vi "file list - sort.vi"(10 "temperature array IN":dbl[](array[numeric]), 11 "path array IN":T1[](array[typedef])) -> (0 "timestamp OUT":dbl[](array[numeric]), 2 "temperatures OUT":dbl[](array[numeric]), 3 "sweep file name array OUT":T1[](array[typedef]))   [LabVIEW 2010]
uses:
  sweep file name.ctl
panel:
  in  "dummy 2":T1={"temperature"=0.0, "temperature str"="", "file path"=path "/snowfall/Users/arcadi/Desktop/Ultrasound/Experiment/YBCO_4/Round1/Sweep12/June_2011/062511/221.16400K_300_3100_001_062511.dat", "last mod"=timestamp(0 s since 1904-01-01), "file name str"="", "mod time(min)"=0.0}
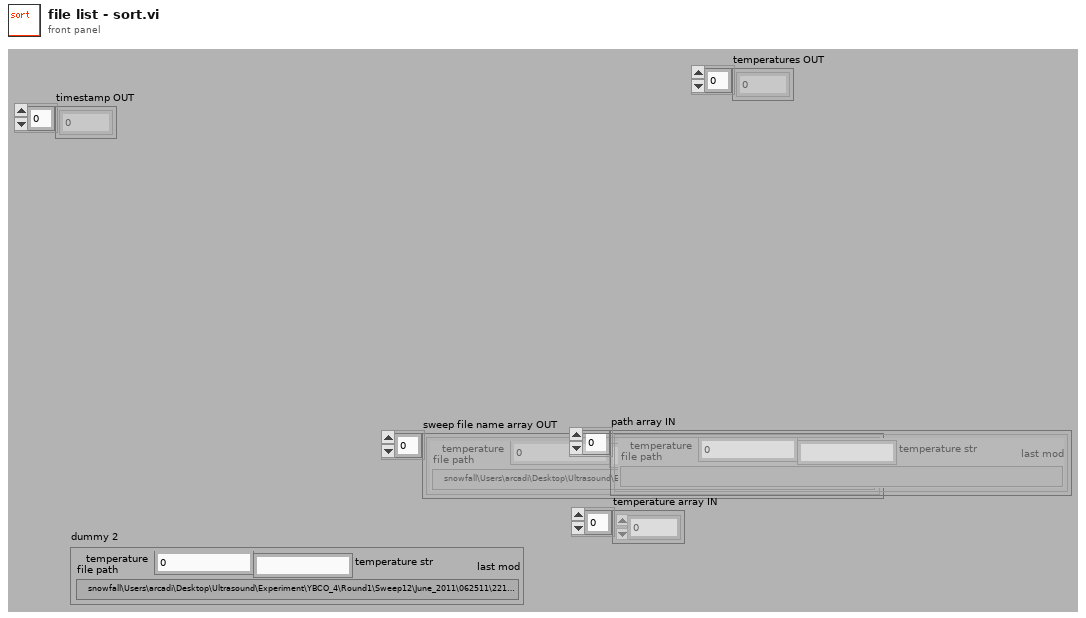
[diagram p1: front panel]
types:
  T1 = typedef "sweep file name.ctl" = cluster{"temperature":dbl, "temperature str":string, "file path":path, "last mod":timestamp, "file name str":string, "mod time(min)":dbl}
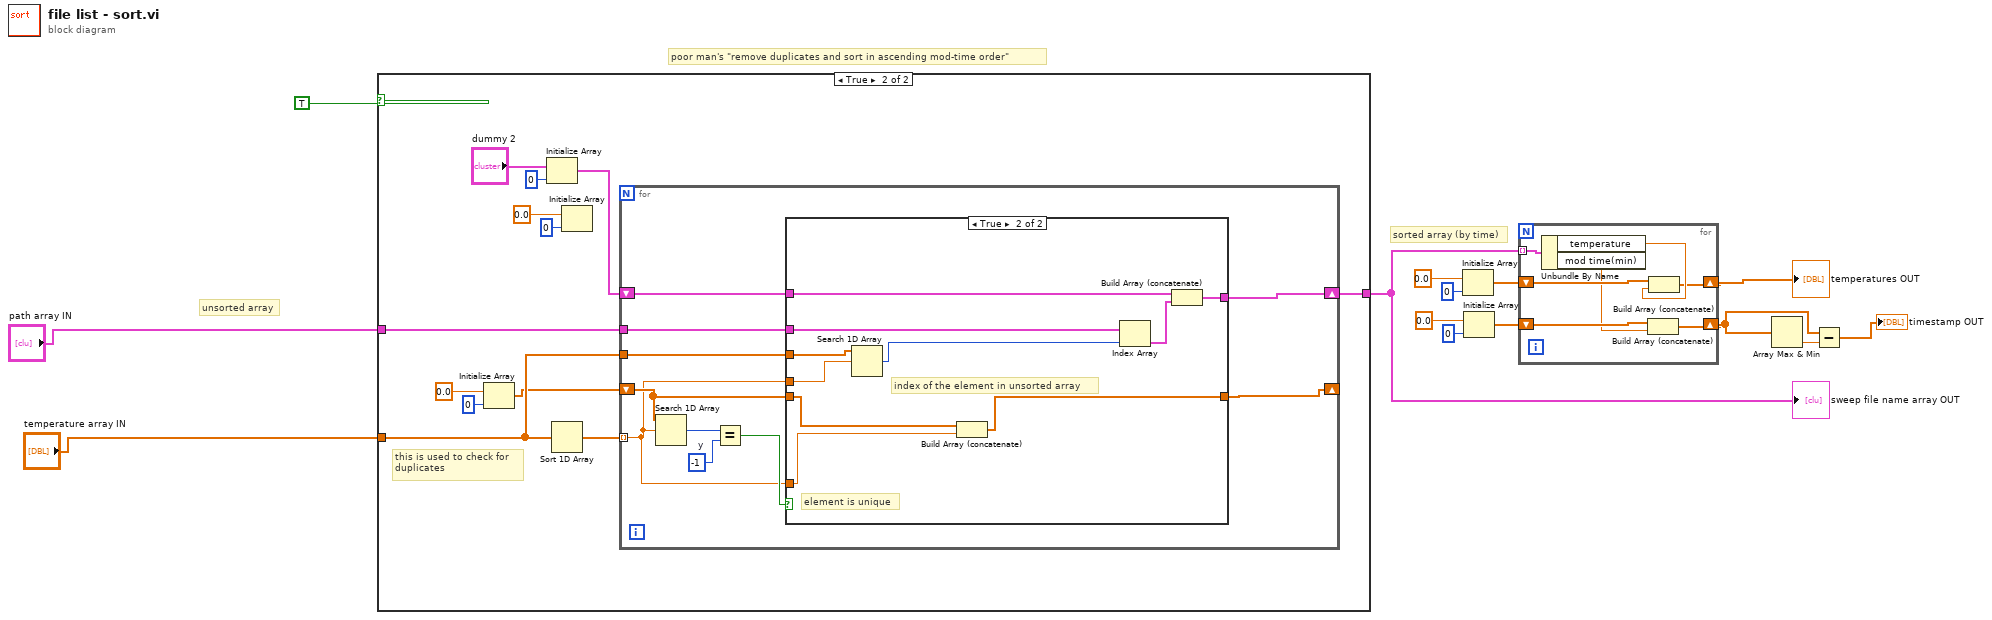
[diagram p0: block diagram]
diagram:
  # "sorted array (by time)"
  # "unsorted array"
  # "poor man's \"remove duplicates and sort in ascending mod-time order\""
  n1 = case shown="True" TRUE {
    tunnel: "temperature array IN" -> [_ w19]
    tunnel: "path array IN" -> [w15 w26]
    tunnel: [w15 w25] -> w3
    frame False {
    }
    frame True {
      # "this is used to check for \nduplicates"
      n2 = Initialize Array(0.0 ("dimension size"), 0 ("dimension size")) -> (w16:dbl[])
      n3 = Initialize Array("dummy 2", 0 ("dimension size")) -> (w20:T1[])
      n4 = Sort 1D Array(array=w19) -> (sorted array=w27:dbl[])
      n5 = Initialize Array(0.0 ("dimension size"), 0 ("dimension size")) -> ()  [unwired: 1 out]
      n6 = for {
        shift-right: [w34] -> w25
        shift-left: w20 -> [w33]
        shift-right: [w32] -> _
        shift-left: w16 -> [w31]
        tunnel: w27 -> [w28] mode=indexing
        tunnel: w19 -> [w30]
        tunnel: w26 -> [w29]
        w36 = -1  # y
        n7 = Search 1D Array(1D array=w31, element=w28) -> (index of element=w37:i32)  [unwired: 1 in]
        n8 = Equal?(x=w37, y=w36) -> (x = y?=w35:bool)
        n9 = case shown="True" w35 {
          tunnel: [w39 w48] -> w34
          tunnel: w33 -> [w39 w49]
          tunnel: [w38 w40] -> w32
          tunnel: w31 -> [w38 w42]
          tunnel: w30 -> [_ w47]
          tunnel: w28 -> [_ w46]
          tunnel: w29 -> [_ w44]
          tunnel: w28 -> [_ w41]
          frame False {
            # "element is not unique"
          }
          frame True {
            # "index of the element in unsorted array"
            # "element is unique"
            n10 = Search 1D Array(1D array=w47, element=w46) -> (index of element=w45:i32)  [unwired: 1 in]
            n11 = Build Array (concatenate)(w42, w41) -> (w40:dbl[])
            n12 = Index Array(array=w44, index=w45) -> (element=w43:T1)
            n13 = Build Array (concatenate)(w49, w43) -> (w48:T1[])
          }
        }
      }
    }
  }
  "sweep file name array OUT" <- w3
  n14 = Initialize Array(0.0 ("dimension size"), 0 ("dimension size")) -> (w10:dbl[])
  n15 = Initialize Array(0.0 ("dimension size"), 0 ("dimension size")) -> (w7:dbl[])
  n16 = for {
    tunnel: w3 -> [w56] mode=indexing
    shift-right: [w50] -> w6
    shift-left: w10 -> [w54]
    shift-right: [w51] -> w5
    shift-left: w7 -> [w53]
    n17 = Unbundle By Name(w56) -> ("temperature"=w55:dbl, "mod time(min)"=w52:dbl)
    n18 = Build Array (concatenate)(w53, w52) -> (w51:dbl[])
    n19 = Build Array (concatenate)(w54, w55) -> (w50:dbl[])
  }
  "temperatures OUT" <- w6
  n20 = Array Max & Min(array=w5) -> (min value=w14:dbl)  [unwired: 3 out]
  n21 = Subtract(x=w5, y=w14) -> (x-y=→"timestamp OUT":dbl[])
